vi "YUYV2RGB.vi"(7 "1D":bool, 8 "col":i32, 9 "row":i32, 10 "Array1D":u8[](array[numeric]), 11 "inputArray":u16[][](array[numeric])) -> (3 "output array":u32[][](array[numeric]))   [LabVIEW 2016]
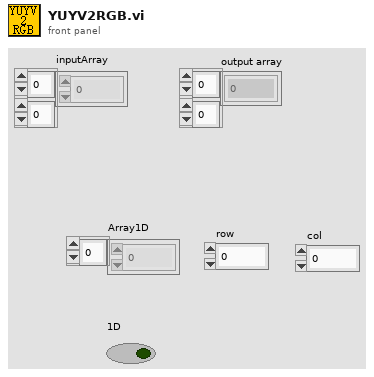
[diagram p1: front panel]
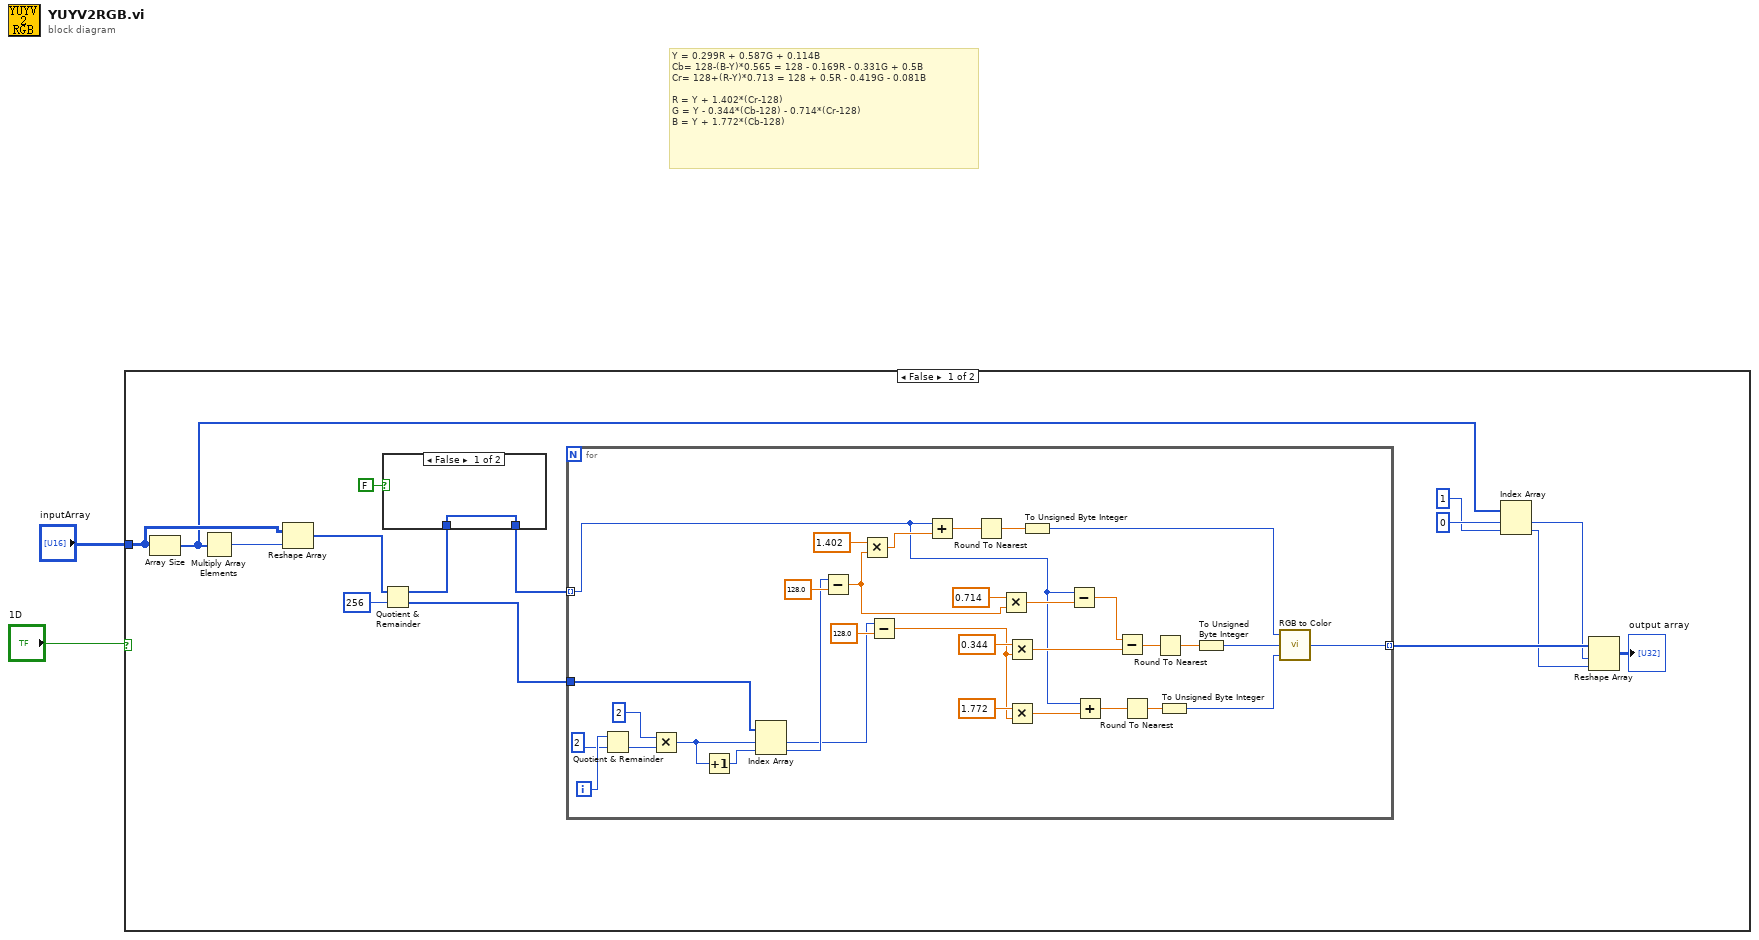
[diagram p0: block diagram]
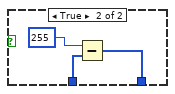
[diagram p2: hidden frame]
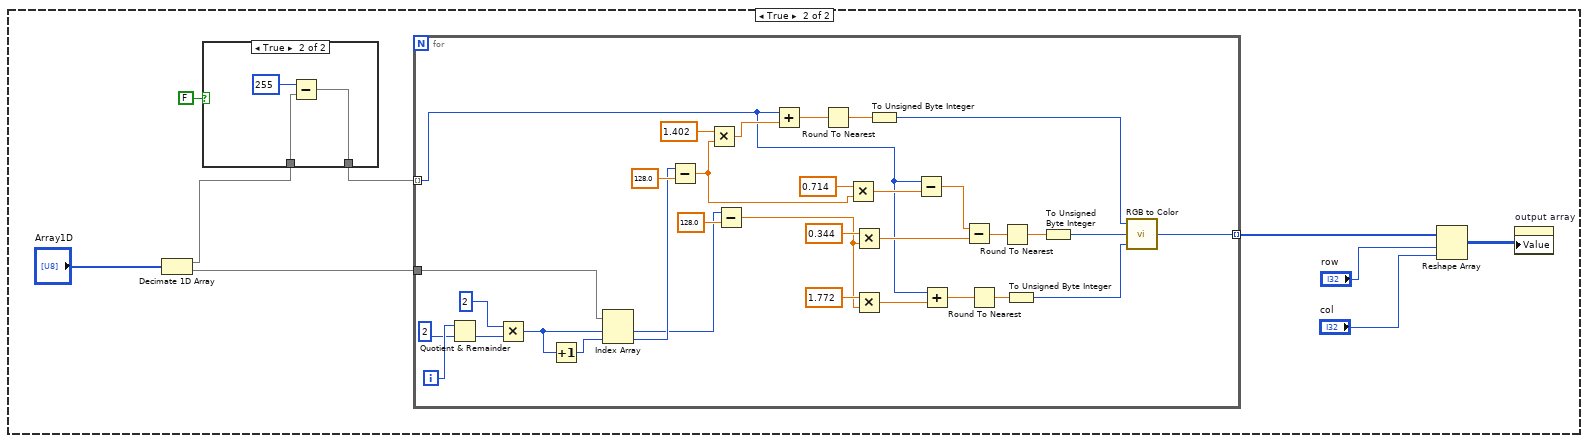
[diagram p3: hidden frame]
diagram:
  # "Y = 0.299R + 0.587G + 0.114B\nCb= 128-(B-Y)*0.565 = 128 - 0.169R - 0.331G + 0.5B\nCr= 128+(R-Y)*0.713 = 128 + 0.5R - 0.419G - 0.081B\n\nR = Y + 1.402*(Cr-128)\nG = Y - 0.344*(Cb-128) - 0.714*(Cr-128)\nB = Y + 1.772*(Cb-128)"
  n1 = case shown="False" "1D" {
    tunnel: "inputArray" -> [w17 _]
    frame False {
      n2 = Array Size(array=w17) -> (size(s)=w12:i32[])
      n3 = Multiply Array Elements(1:w12) -> (0:w16:i32)
      n4 = Reshape Array(w17, w16) -> (w14:u16[])
      n5 = Quotient & Remainder(x=w14, y=u16 256) -> (x-y*floor(x/y)=w5:u16[], floor(x/y)=w13:u16[])
      n6 = case shown="False" FALSE {
        tunnel: w5 -> [w18 w20]
        tunnel: [w18 w19] -> w4
        frame False {
        }
        frame True {
          n7 = Subtract(x=u8 255, y=w20) -> (x-y=w19:u16[])
        }
      }
      n8 = for {
        tunnel: w4 -> [w34] mode=indexing
        tunnel: w13 -> [w52]
        tunnel: [w22] -> w9 mode=indexing
        i -> [w54]
        n9 = Quotient & Remainder(x=w54, y=2) -> (floor(x/y)=w51:i32)  [unwired: 1 out]
        n10 = Multiply(x=2, y=w51) -> (x*y=w33:i32)
        n11 = Increment(x=w33) -> (x+1=w50:i32)
        n12 = Index Array(array=w52, index #1=w33, index #2=w50) -> (element #1=w43:u16, element #2=w47:u16)
        n13 = Subtract(x=w47, y=128.0) -> (x-y=w41:dbl)
        n14 = Multiply(x=1.402, y=w41) -> (x*y=w46:dbl)
        n15 = Subtract(x=w43, y=128.0) -> (x-y=w36:dbl)
        n16 = Add(x=w34, y=w46) -> (x+y=w31:dbl)
        n17 = Round To Nearest(number=w31) -> (nearest integer value=w28:dbl)
        n18 = Multiply(x=0.714, y=w41) -> (x*y=w40:dbl)
        n19 = Multiply(x=0.344, y=w36) -> (x*y=w38:dbl)
        n20 = Multiply(x=1.772, y=w36) -> (x*y=w35:dbl)
        n21 = To Unsigned Byte Integer(number=w28) -> (unsigned 8bit integer=w25:u8)
        n22 = Subtract(x=w34, y=w40) -> (x-y=w39:dbl)
        n23 = Add(x=w34, y=w35) -> (x+y=w30:dbl)
        n24 = Subtract(x=w39, y=w38) -> (x-y=w29:dbl)
        n25 = Round To Nearest(number=w30) -> (nearest integer value=w26:dbl)
        n26 = Round To Nearest(number=w29) -> (nearest integer value=w27:dbl)
        n27 = To Unsigned Byte Integer(number=w26) -> (unsigned 8bit integer=w23:u8)
        n28 = To Unsigned Byte Integer(number=w27) -> (unsigned 8bit integer=w24:u8)
        n29 = call <vilib>:"RGB to Color.vi"("B"=w23, "G"=w24, "R"=w25) -> ("Color"=w22:u32)
      }
      n30 = Index Array(array=w12, index #1=0 ("index"), index #2=1 ("index")) -> (element #1=w8:i32, element #2=w7:i32)
      n31 = Reshape Array(w9, w8, w7) -> (→"output array":u32[][])
    }
    frame True {
      n32 = Decimate 1D Array("Array1D") -> (w57:u8[], w62:u8[])
      n33 = case shown="True" FALSE {
        tunnel: w57 -> [w64 w66]
        tunnel: [w64 w65] -> w56
        frame False {
        }
        frame True {
          n34 = Subtract(x=u8 255, y=w66) -> (x-y=w65:u8[])
        }
      }
      n35 = for {
        tunnel: w56 -> [w80] mode=indexing
        tunnel: w62 -> [w98]
        tunnel: [w68] -> w61 mode=indexing
        i -> [w100]
        n36 = Quotient & Remainder(x=w100, y=2) -> (floor(x/y)=w97:i32)  [unwired: 1 out]
        n37 = Multiply(x=2, y=w97) -> (x*y=w79:i32)
        n38 = Increment(x=w79) -> (x+1=w96:i32)
        n39 = Index Array(array=w98, index #1=w79, index #2=w96) -> (element #1=w89:u8, element #2=w93:u8)
        n40 = Subtract(x=w93, y=128.0) -> (x-y=w87:dbl)
        n41 = Multiply(x=1.402, y=w87) -> (x*y=w92:dbl)
        n42 = Subtract(x=w89, y=128.0) -> (x-y=w82:dbl)
        n43 = Add(x=w80, y=w92) -> (x+y=w77:dbl)
        n44 = Round To Nearest(number=w77) -> (nearest integer value=w74:dbl)
        n45 = Multiply(x=0.714, y=w87) -> (x*y=w86:dbl)
        n46 = Multiply(x=0.344, y=w82) -> (x*y=w84:dbl)
        n47 = Multiply(x=1.772, y=w82) -> (x*y=w81:dbl)
        n48 = To Unsigned Byte Integer(number=w74) -> (unsigned 8bit integer=w71:u8)
        n49 = Subtract(x=w80, y=w86) -> (x-y=w85:dbl)
        n50 = Add(x=w80, y=w81) -> (x+y=w76:dbl)
        n51 = Subtract(x=w85, y=w84) -> (x-y=w75:dbl)
        n52 = Round To Nearest(number=w76) -> (nearest integer value=w72:dbl)
        n53 = Round To Nearest(number=w75) -> (nearest integer value=w73:dbl)
        n54 = To Unsigned Byte Integer(number=w72) -> (unsigned 8bit integer=w69:u8)
        n55 = To Unsigned Byte Integer(number=w73) -> (unsigned 8bit integer=w70:u8)
        n56 = call <vilib>:"RGB to Color.vi"("B"=w69, "G"=w70, "R"=w71) -> ("Color"=w68:u32)
      }
      n57 = Reshape Array(w61, "row", "col") -> (w58:u32[][])
      n58 = property on="output array" class="Arr (strict)"("Value"=w58) -> ()  [unwired: 2 in, 2 out]
    }
  }
